vi "CRYSet basic format Front Panel.vi"(11 "Vi Ref":refnum<vi>) -> ()   [LabVIEW 2013]
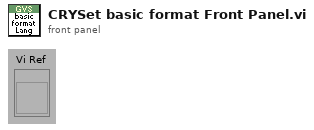
[diagram p1: front panel]
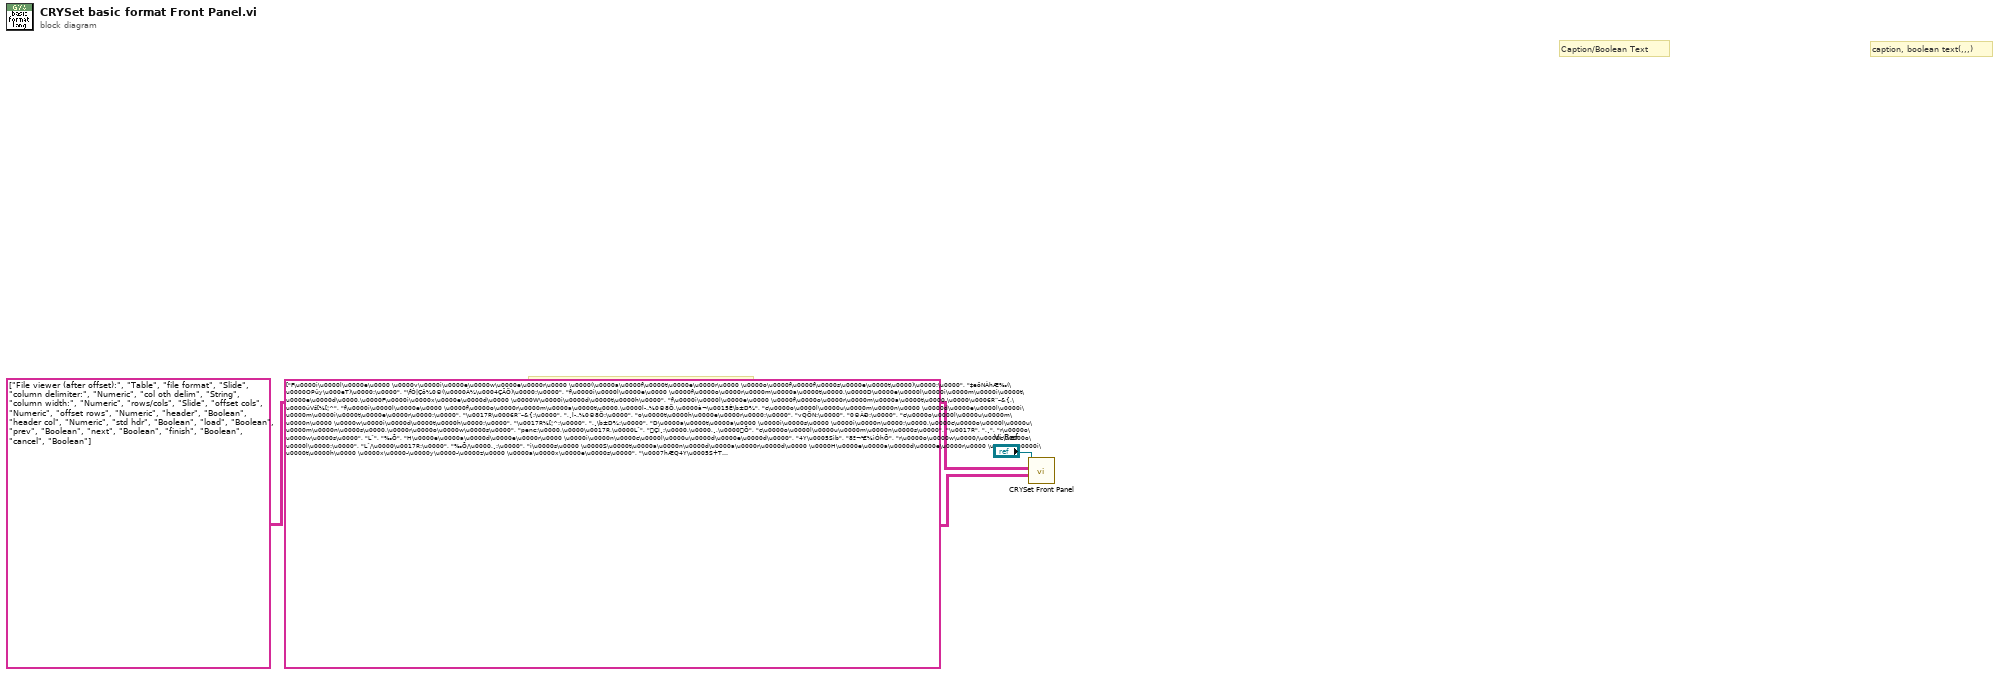
[diagram p0: block diagram]
diagram:
  # "Caption, Tab Page, Multilist Header, Button 4"
  # "Control Type"
  # "Control Name and Tab"
  # "caption, boolean text(,,,)"
  # "Caption/Boolean Text"
  n1 = call "CRYSet Front Panel.vi"("Caption(Boolean Text)"=string[][] [["F\u0000i\u0000l\u0000e\u0000 \u0000v\u0000i\u0000e\u0000w\u0000e\u0000r\u0000 \u0000(\u0000a\u0000f\u0000t\u0000e\u0000r\u0000 \u0000o\u0000f\u0000f\u0000s\u0000e\u0000t\u0000)\u0000:\u0000", "‡eöNÀhÆ‰(\u0000OPûy\u000eT)\u0000:\u0000", "\fÓ|Çô¼0®(\u0000À¼\u0004ÇÄÖ)\u0000:\u0000"], ["f\u0000i\u0000l\u0000e\u0000 \u0000f\u0000o\u0000r\u0000m\u0000a\u0000t\u0000,\u0000D\u0000e\u0000l\u0000i\u0000m\u0000i\u0000t\u0000e\u0000d\u0000,\u0000F\u0000i\u0000x\u0000e\u0000d\u0000 \u0000W\u0000i\u0000d\u0000t\u0000h\u0000", "f\u0000i\u0000l\u0000e\u0000 \u0000f\u0000o\u0000r\u0000m\u0000a\u0000t\u0000,\u0000\u0006R”–&{,\u0000úVš[½[¦^", "f\u0000i\u0000l\u0000e\u0000 \u0000f\u0000o\u0000r\u0000m\u0000a\u0000t\u0000,\u0000l­„½0®8Ö,\u0000à¬\u0015È\b±D¾"], ["c\u0000o\u0000l\u0000u\u0000m\u0000n\u0000 \u0000d\u0000e\u0000l\u0000i\u0000m\u0000i\u0000t\u0000e\u0000r\u0000:\u0000", "\u0017R\u0006R”–&{:\u0000", ",¸l­„½0®8Ö:\u0000"], ["o\u0000t\u0000h\u0000e\u0000r\u0000:\u0000", "vQÖN:\u0000", "0®ÀÐ:\u0000"], ["c\u0000o\u0000l\u0000u\u0000m\u0000n\u0000 \u0000w\u0000i\u0000d\u0000t\u0000h\u0000:\u0000", "\u0017R½[¦^:\u0000", ",¸\b±D¾:\u0000"], ["D\u0000a\u0000t\u0000a\u0000 \u0000i\u0000s\u0000 \u0000i\u0000n\u0000:\u0000,\u0000c\u0000o\u0000l\u0000u\u0000m\u0000n\u0000s\u0000,\u0000r\u0000o\u0000w\u0000s\u0000", "penc:\u0000,\u0000\u0017R,\u0000Lˆ", "ÇÌ¸:\u0000,\u0000,¸,\u0000Õ"], ["c\u0000o\u0000l\u0000u\u0000m\u0000n\u0000s\u0000", "\u0017R", ",¸"], ["r\u0000o\u0000w\u0000s\u0000", "Lˆ", "‰Õ"], ["H\u0000e\u0000a\u0000d\u0000e\u0000r\u0000 \u0000i\u0000n\u0000c\u0000l\u0000u\u0000d\u0000e\u0000d\u0000", "4Y\u0005Sìb", "8º¬¹€½ìÓhÕ"], ["r\u0000o\u0000w\u0000/\u0000c\u0000o\u0000l\u0000:\u0000", "Lˆ/\u0000\u0017R:\u0000", "‰Õ/\u0000,¸:\u0000"], ["i\u0000s\u0000 \u0000S\u0000t\u0000a\u0000n\u0000d\u0000a\u0000r\u0000d\u0000 \u0000H\u0000e\u0000a\u0000d\u0000e\u0000r\u0000 \u0000w\u0000i\u0000t\u0000h\u0000 \u0000x\u0000-\u0000y\u0000-\u0000z\u0000 \u0000a\u0000x\u0000e\u0000s\u0000", "\u0007hÆQ4Y\u0005S+Tt", "•ÍtÇ \u0000ˆÇ”² \u0000\\Ô\u0000É8º¬¹€½"], ["L\u0000o\u0000a\u0000d\u0000 \u0000S\u0000e\u0000t\u0000t\u0000i\u0000n\u0000g\u0000s\u0000.\u0000.\u0000.\u0000", "艌eQ緥n.\u0000.\u0000.\u0000", "\u0015ÖÝÂ\u0001È¬Ç.\u0000.\u0000.\u0000"], ["<\u0000 \u0000P\u0000r\u0000e\u0000v\u0000", "<\u0000\nN\u0000Nek", "<\u0000tÇ\u0004È"], ["N\u0000e\u0000x\u0000t\u0000 \u0000>\u0000", "\u000bN\u0000Nek>\u0000", "ä²LÇ>\u0000"], ["F\u0000i\u0000n\u0000i\u0000s\u0000h\u0000", "Œ[\u0010b", "DÆÌ¸"], ["C\u0000a\u0000n\u0000c\u0000e\u0000l\u0000", "ÖSˆm", "èÍŒÁ"]], "Control ID and Type(Label Name, Type)"=string[][] [["File viewer (after offset):", "Table"], ["file format", "Slide"], ["column delimiter:", "Numeric"], ["col oth delim", "String"], ["column width:", "Numeric"], ["rows/cols", "Slide"], ["offset cols", "Numeric"], ["offset rows", "Numeric"], ["header", "Boolean"], ["header col", "Numeric"], ["std hdr", "Boolean"], ["load", "Boolean"], ["prev", "Boolean"], ["next", "Boolean"], ["finish", "Boolean"], ["cancel", "Boolean"]], "Vi Ref"="Vi Ref") -> ()  [unwired: 9 in]
